vi "ActDriveStraightWeird.vi"(9 "FirstTime":bool, 10 "MaxSpeed (ft/s)":dbl, 11 "Dist (ft)":dbl) -> (1 "XSpeedDemand":dbl, 3 "Done":bool)   [LabVIEW 2020]
doc: "Robot will drive forward straight a set distance utilizing position control \n\nInputs:\n-- MaxSpeed -- Double -- in ft/s, the MaxSpeed the robot can go -- \n-- Dist (ft) -- Double -- Distance in feet you want the robot to go -- \n-- FirstTime -- Boolean -- Input true the first time this function is called, sets the target position -- \n\nOutputs:\n-- Done -- Bool -- has the robot reached its target distance\n-- LeftSpeedDemand -- Double -- Speed Demand for left drive train inorder to reach target -- \n-- RightSpeedDemand -- Double -- Speed Demand for left drive train inorder to reach target --"
uses:
  <vilib>/Rock Robotics/WPI/ThirdParty/JAS_Junk/TrajLib/Trajectory_Library.lvlib
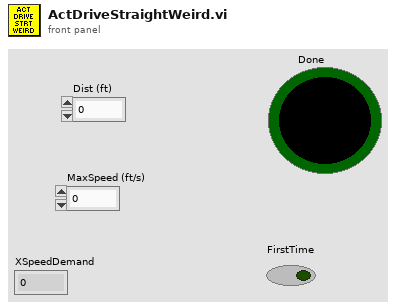
[diagram p1: front panel]
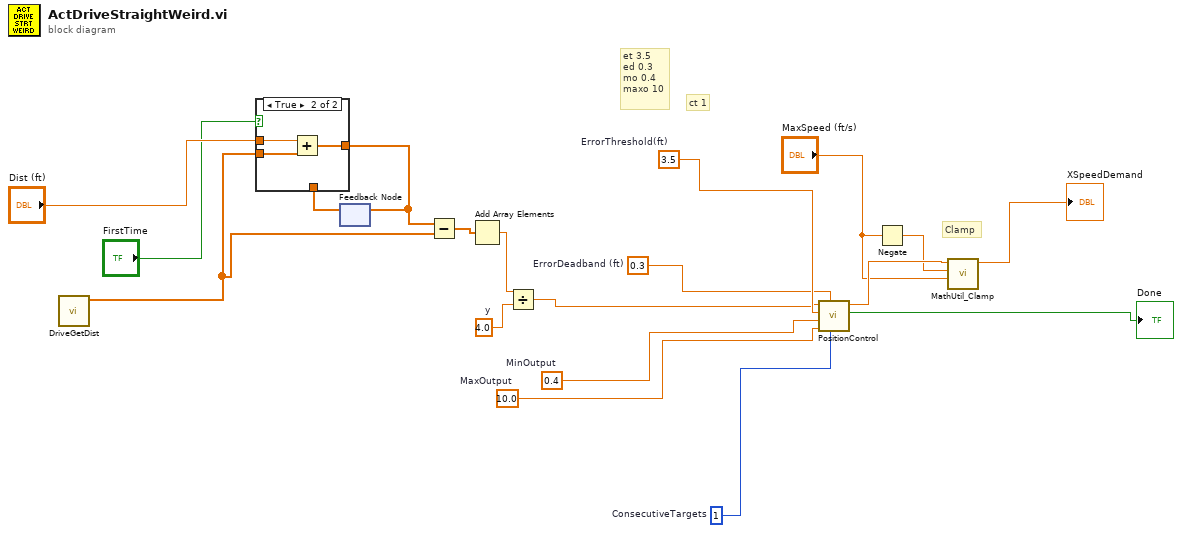
[diagram p0: block diagram]
diagram:
  w14 = 4.0  # y
  w6 = 10.0  # MaxOutput
  w5 = 0.4  # MinOutput
  w7 = 1  # ConsecutiveTargets
  w2 = 0.3  # ErrorDeadband (ft)
  w4 = 3.5  # ErrorThreshold(ft)
  # "Clamp"
  # "ct 1"
  # "et 3.5\ned 0.3\nmo 0.4\nmaxo 10"
  n1 = call "DriveGetDist.vi"() -> ("ModuleTravelPosition"=w15:dbl[])  [unwired: 11 in]
  n2 = feedback #1() -> (w18:dbl[])  [unwired: 1 in]
  n3 = case shown="True" "FirstTime" {
    tunnel: "Dist (ft)" -> [_ w23]
    tunnel: [w20 w22] -> w17
    tunnel: w18 -> [w20 _]
    tunnel: w15 -> [_ w21]
    frame False {
    }
    frame True {
      n4 = Add(x=w23, y=w21) -> (x+y=w22:dbl[])
    }
  }
  n5 = feedback-in #1(w17) -> ()
  n6 = Subtract(x=w17, y=w15) -> (x-y=w13:dbl[])
  n7 = Add Array Elements(numeric array=w13) -> (sum=w12:dbl)
  n8 = Divide(x=w12, y=w14) -> (x/y=w3:dbl)
  n9 = call "PositionControl.vi"("ConsecutiveTargets"=w7, "ErrorDeadband"=w2, "MaxOutput"=w6, "MinOutput"=w5, "ErrorThreshold"=w4, "Error"=w3) -> ("OnTarget"=→"Done":bool, "OutputValue"=w11:dbl)  [unwired: 3 in, 1 out]
  n10 = Negate(x="MaxSpeed (ft/s)") -> (-x=w10:dbl)
  n11 = call <vilib>:"MathUtil_Clamp.vi"("High Limit"="MaxSpeed (ft/s)", "Low Limit"=w10, "Value"=w11) -> ("Result"=→"XSpeedDemand":dbl)  [unwired: 8 in]
